vi "fgv_system_progress.vi"(7 "cmd":enum16{"read", "write"}(ring), 11 "progress status":T1) -> (3 "progress status out":T1)   [LabVIEW 2019]
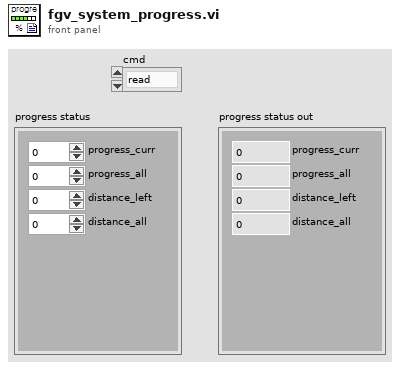
[diagram p1: front panel]
types:
  T1 = cluster{"progress_curr":dbl, "progress_all":dbl, "distance_left":dbl, "distance_all":dbl}
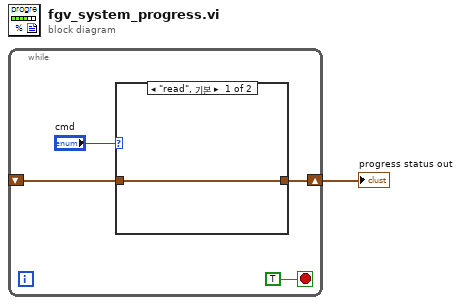
[diagram p0: block diagram]
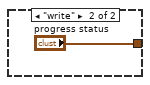
[diagram p2: hidden frame]
diagram:
  n1 = while {
    shift-right: [w3] -> w1
    shift-left: _ -> [w2]
    stop <- TRUE stop-if-true
    n2 = case shown="\"read\", 기본" "cmd" {
      tunnel: [w6 "progress status"] -> w3
      tunnel: w2 -> [w6 _]
      frame "read", Default {
      }
      frame "write" {
      }
    }
  }
  "progress status out" <- w1
